vi "ObstacleAvoid.vi"(3 "SupressIn":dbl, 7 "Inhibit":bool, 8 "HowAmI? Clean":cluster{"T":dbl, "Battery":dbl, "Temp":dbl}, 9 "WhatAroundMe? Clean":cluster{"T":dbl, "Range":dbl, "Bearing":dbl}[](array[cluster]), 10 "WhereAmI? Clean":T1, 11 "VelCom":dbl) -> (0 "SupressOut":dbl, 2 "ActCommand":dbl[](array[numeric]))   [LabVIEW 2011]
doc: "This behavior takes in the What is around me? data and produces an output velocity array using two rules:\n1) if the range at any bearing is greater that the collison range, pass on the current commanded velocity form the Forebrain.\n2) if the range is less at any bearing, pass on a velocity calculated by the follwing formla:\n\n Vel=(VelCom/collisionstandoff)*Range-k*VelCom where k=slow down scale factor.\n\nThis obstacle avoidance behavior will slow the robot down when approaching an obstacle and eventually stop it before hitting the obstacel.\n\nIt is designed to work with a 90 element behavior arbiter."
uses:
  WhereAmI.ctl
panel:
  # "This sub VI converts the What is around me? data into an obstacle avoidance velocity array"
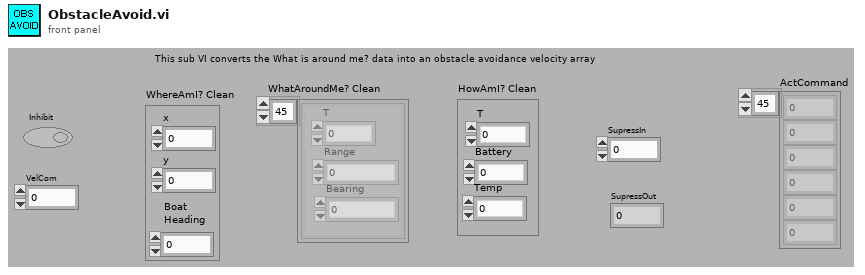
[diagram p1: front panel]
types:
  T1 = typedef "WhereAmI.ctl" = cluster{"x":sgl, "y":sgl, "Boat\nHeading":sgl}
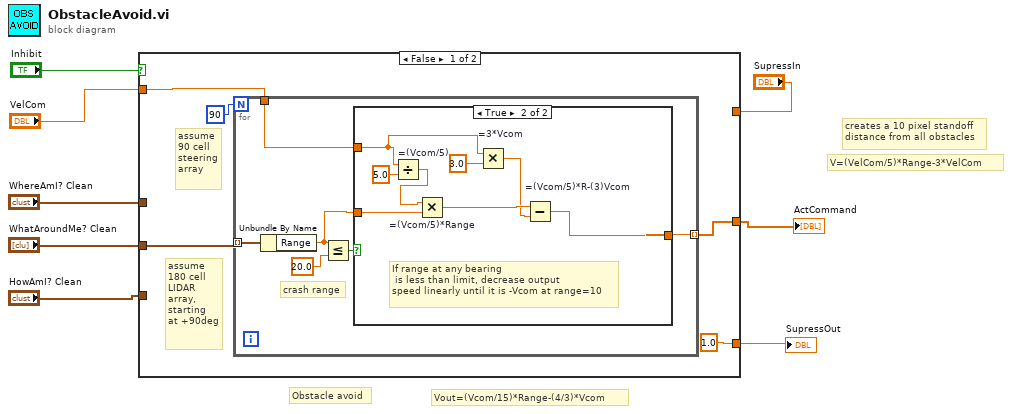
[diagram p0: block diagram]
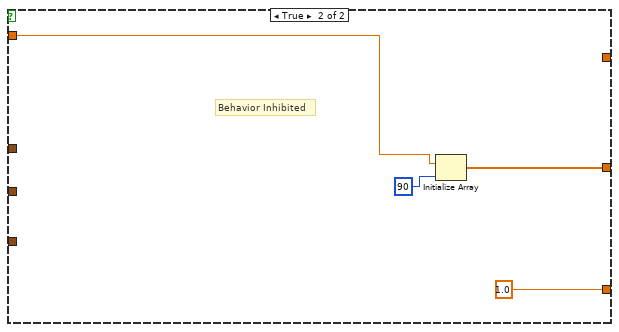
[diagram p3: hidden frame]
diagram:
  # "V=(VelCom/5)*Range-3*VelCom"
  # "creates a 10 pixel standoff \ndistance from all obstacles"
  # "Vout=(Vcom/15)*Range-(4/3)*Vcom"
  # "Obstacle avoid"
  n1 = case shown="False" "Inhibit" {
    tunnel: "VelCom" -> [w11 w29]
    tunnel: "WhatAroundMe? Clean" -> [w12 _]
    tunnel: "WhereAmI? Clean" -> [_ _]
    tunnel: "HowAmI? Clean" -> [_ _]
    tunnel: "SupressIn" -> [_ _]
    tunnel: [w9 w30] -> w1
    tunnel: [1.0 ("SupressOut") 1.0 ("SupressOut")] -> w2
    frame False {
      # "assume\n180 cell\nLIDAR\narray,\nstarting\nat +90deg"
      # "assume\n90 cell\nsteering\narray"
      n2 = for {
        N: 90 -> [_]
        tunnel: w12 -> [w19] mode=indexing
        tunnel: w11 -> [w16]
        tunnel: [w14] -> w9 mode=indexing
        # "crash range"
        n3 = Unbundle By Name(w19) -> ("Range"=w15:dbl)
        n4 = Less Or Equal?(x=w15, y=20.0) -> (x <= y?=w18:bool)
        n5 = case shown="True" w18 {
          tunnel: w16 -> [w20 w23]
          tunnel: [w20 w25] -> w14
          tunnel: w15 -> [_ w24]
          frame False {
            # "if range > 20\nat any bearing\nJust pass speed on"
          }
          frame True {
            # "If range at any bearing\n is less than limit, decrease output\nspeed linearly until it is -Vcom at range=10"
            n6 = Divide "=(Vcom/5)"(x=w23, y=5.0) -> (x/y=w27:dbl)
            n7 = Multiply "=(Vcom/5)*Range"(x=w27, y=w24) -> (x*y=w26:dbl)
            n8 = Multiply "=3*Vcom"(x=w23, y=3.0) -> (x*y=w21:dbl)
            n9 = Subtract "=(Vcom/5)*R-(3)Vcom"(x=w26, y=w21) -> (x-y=w25:dbl)
          }
        }
      }
    }
    frame True {
      # "Behavior Inhibited"
      n10 = Initialize Array "Initialize Array"(w29, 90 ("dimension size")) -> (w30:dbl[])
    }
  }
  "ActCommand" <- w1
  "SupressOut" <- w2
